vi "Stepper Set Zero.vi"(1 "error in (no error)":errorcluster, 2 "Motor Number":u32=1 min=1 max=255 step=1, 3 "Instrument Address":refnum<visa-resource-name>) -> (0 "error out":errorcluster)   [LabVIEW 2020]
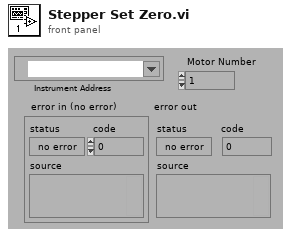
[diagram p1: front panel]
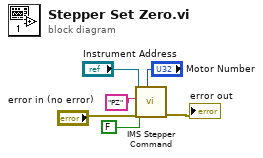
[diagram p0: block diagram]
diagram:
  n1 = call "IMS Stepper Command.vi"("Motor Number"="Motor Number", "error in (no error)"="error in (no error)", "Mode"=FALSE, "Command"="PZ", "Instrument Address"="Instrument Address") -> ("error out"=→"error out":errorcluster)  [unwired: 1 in, 3 out]
